vi "Loadcfg_writeslaveP.vi"(8 "error in":errorcluster, 11 "Data Cluster in":T2) -> (0 "error out":errorcluster, 3 "Data Cluster out":T2)   [LabVIEW 2017, in "Akwizycja.lvlib"]
uses:
  Akwizycja.lvlib
  <vilib>/Plasmionique/MB Master/MB_Master_Serial/MB_Master_Serial.lvclass
  D:/Program Files (x86)/National Instruments/LabVIEW 2017/vi.lib/Plasmionique/MB Master/MB_Master/MB_Master.lvclass
  <vilib>/Plasmionique/MB Master/MB Master.lvlib
  <vilib>/Utility/config.llb/NI_LVConfig.lvlib
panel:
  in  "Px":T1
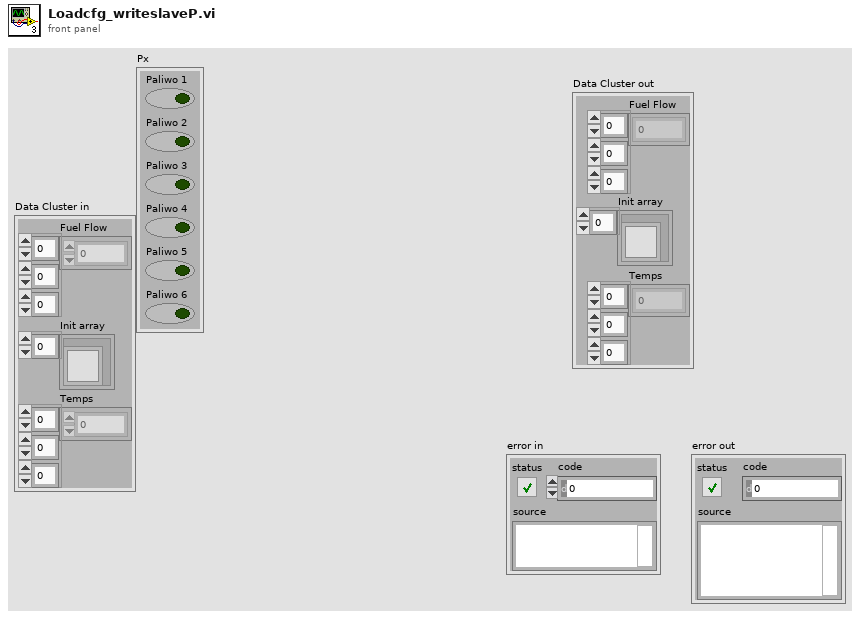
[diagram p1: front panel]
types:
  T1 = cluster{"Paliwo 1":bool, "Paliwo 2":bool, "Paliwo 3":bool, "Paliwo 4":bool, "Paliwo 5":bool, "Paliwo 6":bool}
  T2 = cluster{"Fuel Flow":dbl[][][], "Init array":refnum<class "MB_Master_Serial.lvclass">[], "Temps":dbl[][][]}
  T3 = typedef "NI_LVConfig.lvlib/Config Data RefNum.ctl" = refnum<k1>
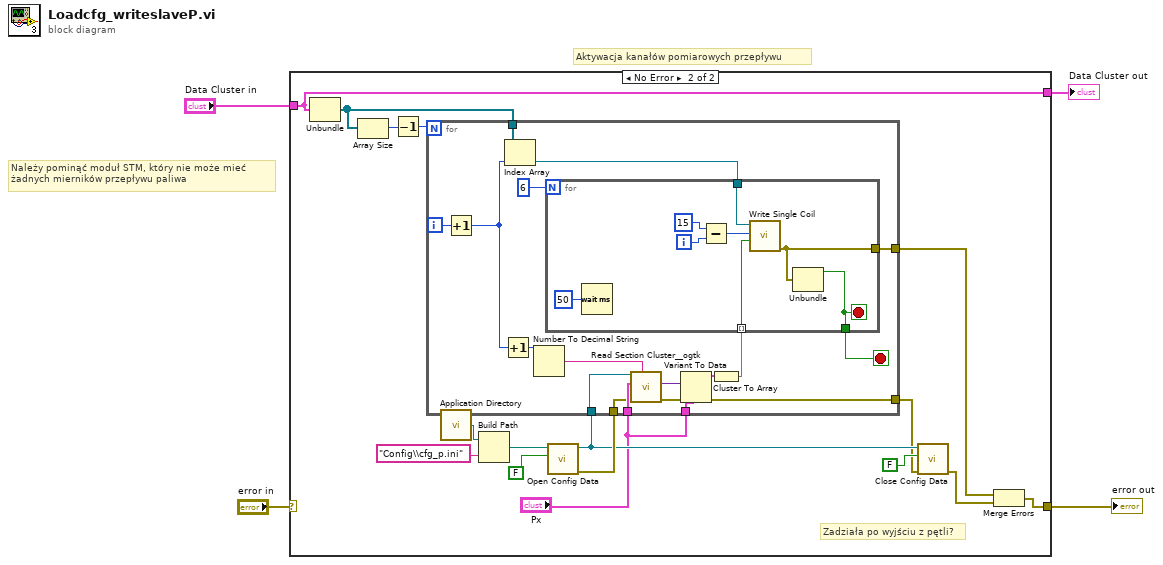
[diagram p0: block diagram]
diagram:
  # "Aktywacja kanałów pomiarowych przepływu"
  # "Należy pominąć moduł STM, który nie może mieć\nżadnych mierników przepływu paliwa"
  # "Należy pominąć moduł STM, który nie może mieć\nżadnych mierników przepływu paliwa"
  n1 = case shown="No Error" "error in" {
    selector: "error in" -> [w6 _]
    tunnel: [w6 w18] -> w4
    tunnel: "Data Cluster in" -> [w5 w9]
    tunnel: [w5 w9] -> w1
    frame Error {
    }
    frame No Error {
      # "Zadziała po wyjściu z pętli?"
      n2 = Unbundle(w9) -> ("Init array"=w8:refnum<class "MB_Master_Serial.lvclass">[])  [unwired: 2 out]
      n3 = Array Size(array=w8) -> (size(s)=w16:i32)
      n4 = Decrement(x=w16) -> (x-1=w15:i32)
      n5 = call <vilib>:"Application Directory.vi"() -> ("Application Directory"=w19:path)
      n6 = Build Path(base path=w19, name or relative path="Config\\cfg_p.ini") -> (appended path=w21:path)
      n7 = call <vilib>:"Open Config Data.vi"("create file if necessary (T)"=FALSE, "configuration file path"=w21) -> ("error out"=w17:errorcluster, "refnum"=w13:T3)  [unwired: 7 in, 1 out]
      n8 = for {
        N: w15 -> [_]
        tunnel: w13 -> [w40]
        tunnel: [w38] -> w11
        tunnel: w8 -> [w30]
        tunnel: [w34] -> w14
        tunnel: "Px" -> [w29]
        tunnel: "Px" -> [w28]
        tunnel: w17 -> [w27]
        i -> [w25]
        stop <- w32 stop-if-true
        n9 = Increment(x=w25) -> (x+1=w24:i32)
        n10 = Increment(x=w24) -> (x+1=w23:i32)
        n11 = Index Array(array=w30, index=w24) -> (element=w31:refnum<class "MB_Master_Serial.lvclass">)
        n12 = Number To Decimal String(number=w23) -> (decimal integer string=w26:string)  [unwired: 1 in]
        n13 = call <userlib>:"Read Section Cluster__ogtk.vi"("section (optional)"=w26, "error in (no error)"=w27, "Section Formatted Cluster Type"=w29, "refnum"=w40) -> ("error out"=w39:errorcluster, "Section Formatted Cluster"=w37:variant)  [unwired: 3 in, 3 out]
        n14 = Variant To Data(error in=w39, type=w28, Variant=w37) -> (data=w36:T1, error out=w38:errorcluster)
        n15 = Cluster To Array(cluster=w36) -> (array=w33:bool[])
        n16 = for {
          N: 6 ("Numeric Control") -> [_]
          tunnel: w31 -> [w46]
          tunnel: [w47] -> w34
          tunnel: w33 -> [w48] mode=indexing
          tunnel: [w45] -> w32
          i -> [w43]
          stop <- w45 stop-if-true
          n17 = Wait (ms)(milliseconds to wait=u32 50) -> ()  [unwired: 1 out]
          n18 = Subtract(x=i8 15, y=w43) -> (x-y=w42:i32)
          n19 = call <vilib>:"Write Single Coil.vi"("value"=w48, "address"=w42, "MB session in"=w46) -> ("error out"=w47:errorcluster)  [unwired: 7 in, 1 out]
          n20 = Unbundle(w47) -> ("status"=w45:bool)  [unwired: 2 out]
        }
      }
      n21 = call <vilib>:"Close Config Data.vi"("error in (no error)"=w11, "write file if changed (T)"=FALSE, "refnum"=w13) -> ("error out"=w10:errorcluster)  [unwired: 7 in, 1 out]
      n22 = Merge Errors(w14, w10) -> (w18:errorcluster)
    }
  }
  "error out" <- w4
  "Data Cluster out" <- w1
